vi "StarMsg.vi"(2 "Bar Value":dbl, 3 "error in (no error)":errorcluster, 4 "Show":bool=TRUE, 5 "Cancel Button (True)":bool=TRUE, 6 "Max Value (100)":dbl=100.0) -> (8 "Cancel":bool, 10 "error out":errorcluster)   [LabVIEW 2014]
doc: "Displays a dialog box complete with a progress bar and cancel button.\n\nThis VI should be called from within a loop with the \"Show\" input set to TRUE, and when the loop exists this VI should be called with \"Show\" set to FALSE."
panel:
  out "Slide":dbl(slide) scale=0.0..100.0
  in  "Cancel Button":bool
  out "String":string
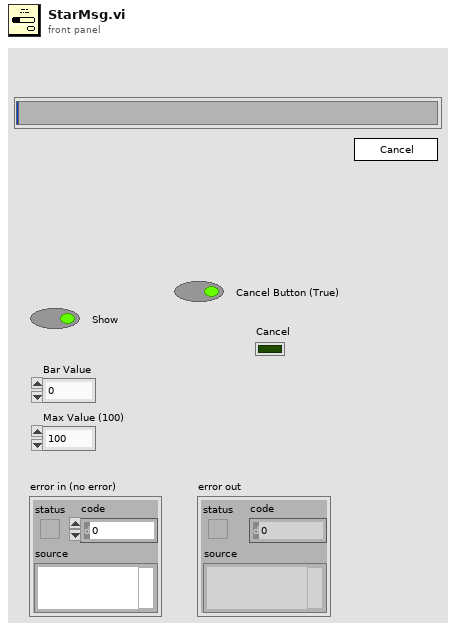
[diagram p1: front panel]
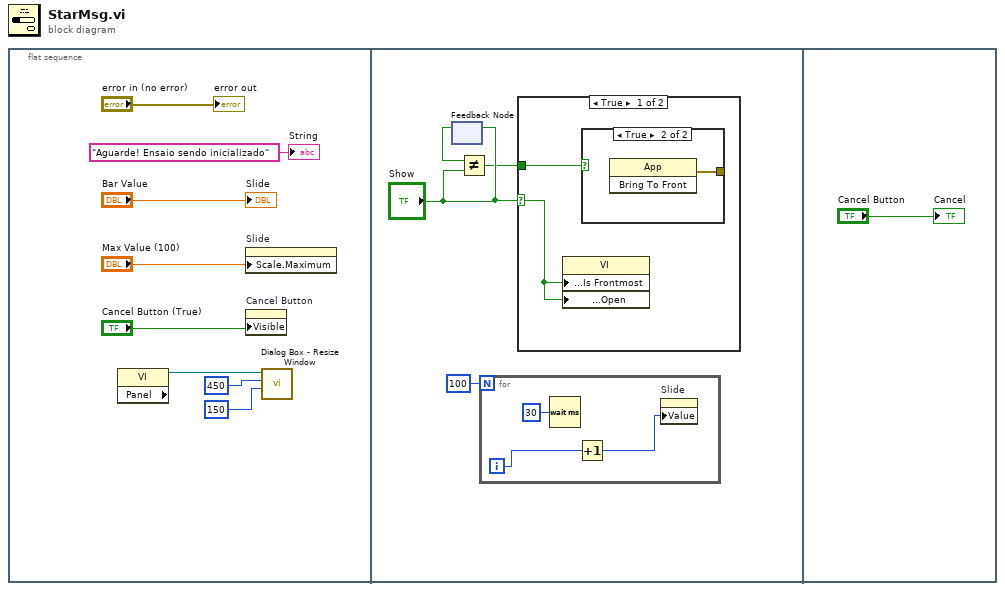
[diagram p0: block diagram]
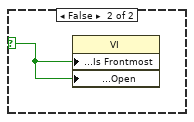
[diagram p3: hidden frame]
diagram:
  n1 = flat-sequence {
    frame #0 {
      n2 = property class="VI" props=["Panel"]() -> (reference out=w4:refnum<vi>)  [unwired: 2 in, 2 out]
      n3 = property on="Slide" class="Slide (strict)"("Scale.Maximum"="Max Value (100)") -> ()  [unwired: 2 in, 2 out]
      n4 = property on="Cancel Button" class="Bool"("Visible"="Cancel Button (True)") -> ()  [unwired: 2 in, 2 out]
      n5 = call "Dialog Box - Resize Window.vi"("Height"=i16 150, "Width"=i16 450, "reference"=w4) -> ()  [unwired: 8 in, 1 out]
      "String" <- "Aguarde! Ensaio sendo inicializado" ("String")
      "error out" <- "error in (no error)"
      "Slide" <- "Bar Value"
    }
    frame #1 {
      n6 = feedback-in #1("Show") -> ()
      n7 = feedback #1() -> (w11:bool)  [unwired: 1 in]
      n8 = Not Equal?(x=w11, y="Show") -> (x != y?=w10:bool)
      n9 = for {
        N: 100 -> [_]
        i -> [w15]
        n10 = Wait (ms)(milliseconds to wait=u32 30) -> ()  [unwired: 1 out]
        n11 = Increment(x=w15) -> (x+1=w14:i32)
        n12 = property on="Slide" class="Slide (strict)"("Value"=w14) -> ()  [unwired: 2 in, 2 out]
      }
      n13 = case shown="True" "Show" {
        selector: "Show" -> [w17 w19]
        tunnel: w10 -> [w16 _]
        frame True {
          n14 = property class="VI"("Front Panel Window:Is Frontmost"=w17, "Front Panel Window:Open"=w17) -> ()  [unwired: 2 in, 2 out]
          n15 = case shown="True" w16 {
            tunnel: [_ w18] -> _
            frame False {
            }
            frame True {
              n16 = invoke class="App" method="Bring To Front"() -> (error out=w18:errorcluster)  [unwired: 3 in, 2 out]
            }
          }
        }
        frame False {
          n17 = property class="VI"("Front Panel Window:Is Frontmost"=w19, "Front Panel Window:Open"=w19) -> ()  [unwired: 2 in, 2 out]
        }
      }
    }
    frame #2 {
      "Cancel" <- "Cancel Button"
    }
  }
